vi "Write Dependencies Properties.vi"(8 "Error In":errorcluster, 10 "All Dependencies Properties":T1[](array[typedef]), 11 "Custom Device .NET Ref In":refnum<k24>) -> (0 "Error Out":errorcluster, 3 "Custom Device .NET Ref Out":refnum<k24>)   [LabVIEW 2015, in "VeriStand Custom Device XML Parser.lvlib"]
doc: "Sets the properties of the dependencies of the custom device"
uses:
  VeriStand Custom Device XML Parser.lvlib
  XML Controls/Dependencies Properties.ctl
  XML Controls/Path Cluster.ctl
  XML Controls/Supported Targets.ctl
  NationalInstruments.VeriStand.XMLReader
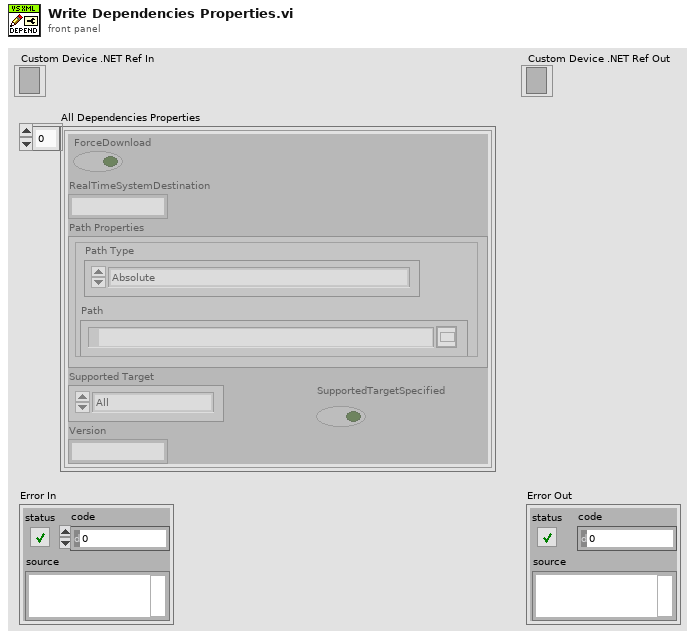
[diagram p1: front panel]
types:
  T1 = typedef "VeriStand Custom Device XML Parser.lvlib/Dependencies Properties.ctl" = cluster{"ForceDownload":bool, "RealTimeSystemDestination":string, "Path Properties":T2, "Supported Target":T3, "Version":string, "SupportedTargetSpecified":bool}
  T2 = typedef "VeriStand Custom Device XML Parser.lvlib/Path Cluster.ctl" = cluster{"Path":path, "Path Type":enum16{"Absolute", "To Base", "To Common Doc Dir", "To Application Data Dir"}}
  T3 = typedef "VeriStand Custom Device XML Parser.lvlib/Supported Targets.ctl" = enum16{"All", "Pharlap", "VxWorks", "Windows", "Linux_32_ARM", "Linux_x64", "PharlapWindows", "PharlapVxWorks", "VxWorksWindows"}
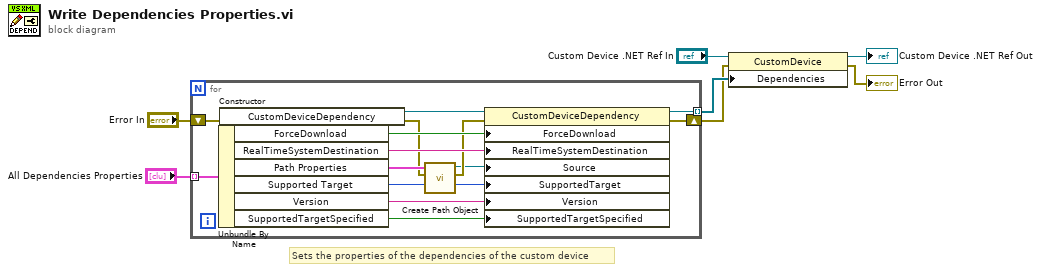
[diagram p0: block diagram]
diagram:
  # "Sets the properties of the dependencies of the custom device"
  n1 = for {
    shift-right: [w11] -> w5
    shift-left: "Error In" -> [w21]
    tunnel: "All Dependencies Properties" -> [w20] mode=indexing
    tunnel: [w10] -> w7 mode=indexing
    n2 = Unbundle By Name(w20) -> ("ForceDownload"=w19:bool, "RealTimeSystemDestination"=w16:string, "Path Properties"=w15:T2, "Supported Target"=w17:T3, "Version"=w18:string, "SupportedTargetSpecified"=w8:bool)
    n3 = constructor class="CustomDeviceDependency"(error in=w21) -> (reference out=w13:refnum<k24>, error out=w14:errorcluster)  [unwired: 2 in, 1 out]
    n4 = call "Create Path Object.vi"("Error In"=w14, "Path Data Cluster"=w15) -> ("Error Out"=w12:errorcluster, "Path .NET Ref"=w9:refnum<k24>)  [unwired: 8 in]
    n5 = property class="CustomDeviceDependency"(reference=w13, error in=w12, "ForceDownload"=w19, "RealTimeSystemDestination"=w16, "Source"=w9, "SupportedTarget"=w17, "Version"=w18, "SupportedTargetSpecified"=w8) -> (reference out=w10:refnum<k24>, error out=w11:errorcluster)
  }
  n6 = property class="CustomDevice"(reference="Custom Device .NET Ref In", error in=w5, "Dependencies"=w7) -> (reference out=→"Custom Device .NET Ref Out":refnum<k24>, error out=→"Error Out":errorcluster)
